vi "SNRPhaseNoiseStructure_ChangePowerFreq.vi"(7 "band":T1 {"stop frequency (Hz)" format="%.2f"; "start frequency (Hz)" format="%.2f"}, 8 "Analyze SNR Input":T2={"Pins"=["Xout"], "Published Data Id"=[], "frequency range"={"start frequency"=-1.0, "stop frequency"=-1.0}}, 9 "RFSG Input":T3={"LO configure setting"={"Carrier Frequency (Hz)"=5180000000.0, "Power Level(dBm)"=-10.0, "External Attenuation (dB)"=0.0}, "Port"=""} {"LO configure setting"."Carrier Frequency (Hz)" format="%#_6p"}, 10 "Scope Input":T4={"Min. Sample Rate"=1000000.0, "Min Record Length"=1000, "Vertical Coupling"=1, "Vertical Range (V)"=2.0, "Pins"=["Xout"]} {"Vertical Range (V)" format="%_3g"; "Vertical Coupling" items=["AC", "DC", "Ground"]; "Min. Sample Rate" format="%#_6p"}, 11 "Semiconductor Module Context":T5) -> (0 "error out":errorcluster)   [LabVIEW 2014]
uses:
  <vilib>/NI_TestStand_SemiconductorModule/NI_TestStand_Semiconductor_Module.lvlibp/PinMap/General/SemiconductorModuleContext.ctl
  Control/Scope Input.ctl
  Control/RFSG Input.ctl
  Control/Digitizier Analyze Input.ctl
  Control/Quene Type_Digitizer.ctl
  <vilib>/NI_TestStand_SemiconductorModule/NI_TestStand_Semiconductor_Module.lvlibp/PinMap/RF/RFPM/PinToNIRFPMSessions.vi
  <vilib>/NI_TestStand_SemiconductorModule/NI_TestStand_Semiconductor_Module.lvlibp
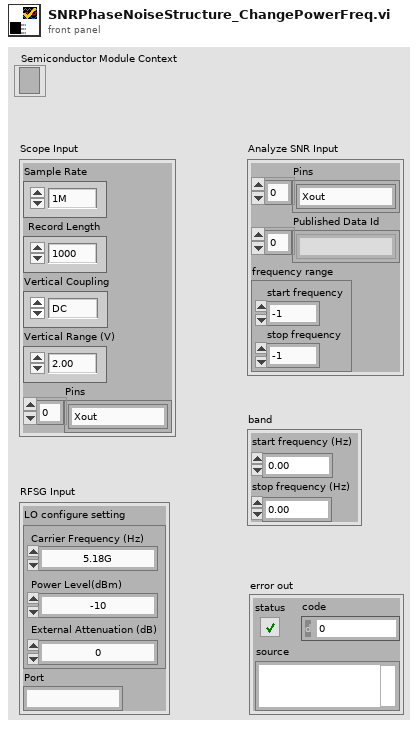
[diagram p1: front panel]
types:
  T1 = cluster{"start frequency (Hz)":dbl, "stop frequency (Hz)":dbl}
  T2 = typedef "Digitizier Analyze Input.ctl" = cluster{"Pins":string[], "Published Data Id":string[], "frequency range":cluster{"start frequency":dbl, "stop frequency":dbl}}
  T3 = typedef "RFSG Input.ctl" = cluster{"LO configure setting":cluster{"Carrier Frequency (Hz)":dbl, "Power Level(dBm)":dbl, "External Attenuation (dB)":dbl}, "Port":string}
  T4 = typedef "Scope Input.ctl" = cluster{"Min. Sample Rate":dbl, "Min Record Length":i32, "Vertical Coupling":i32, "Vertical Range (V)":dbl, "Pins":string[]}
  T5 = typedef "NI_TestStand_Semiconductor_Module.lvlibp/SemiconductorModuleContext.ctl" = refnum<k7>
  T6 = typedef "Quene Type_Digitizer.ctl" = cluster{"Actiion":enum16{"Exit", "Analyze"}, "Waveform Data":waveform(dbl)[], "Semiconductor Module Context":T5, "error constant":errorcluster}
  T7 = cluster{"Carrier Frequency (Hz)":dbl, "Power Level(dBm)":dbl, "External Attenuation (dB)":dbl}
  T8 = cluster{"start frequency":dbl, "stop frequency":dbl}
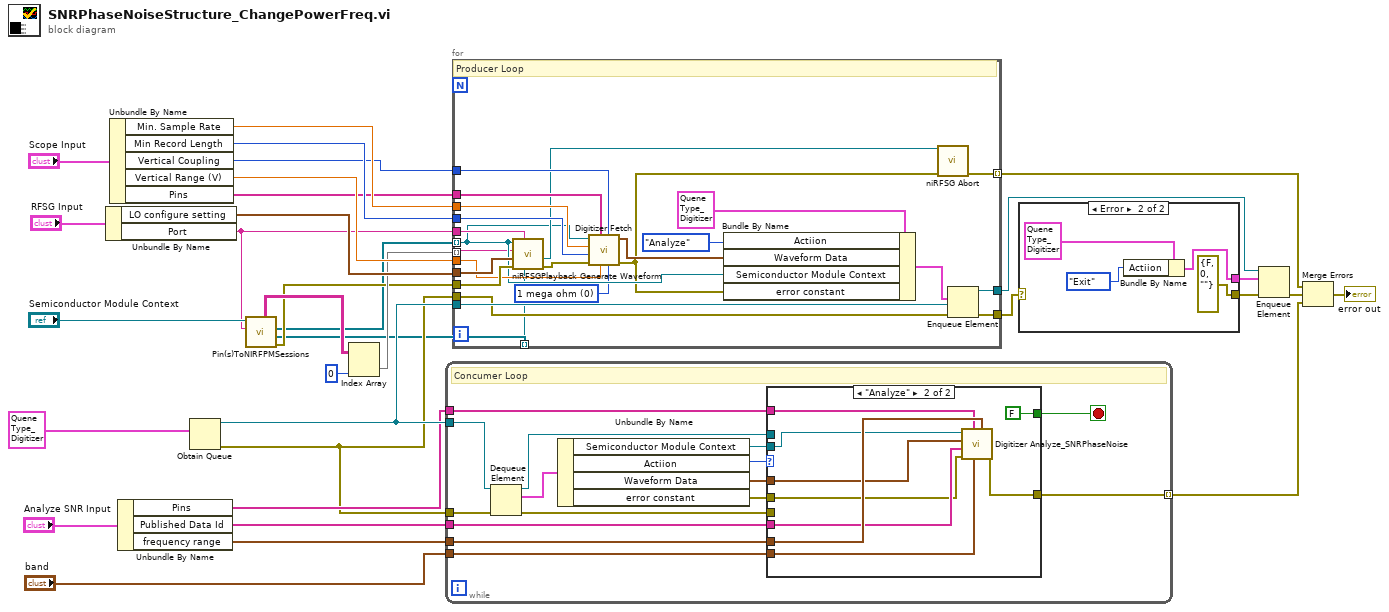
[diagram p0: block diagram]
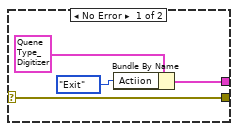
[diagram p2: hidden frame]
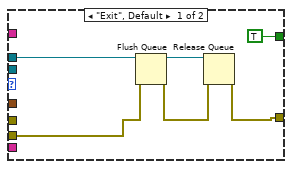
[diagram p3: hidden frame]
diagram:
  n1 = Unbundle By Name("RFSG Input") -> ("LO configure setting"=w30:T7, "Port"=w1:string)
  n2 = Unbundle By Name("Scope Input") -> ("Min. Sample Rate"=w28:dbl, "Min Record Length"=w27:i32, "Vertical Coupling"=w25:i32, "Vertical Range (V)"=w26:dbl, "Pins"=w24:string[])
  n3 = Unbundle By Name("Analyze SNR Input") -> ("Pins"=w18:string[], "Published Data Id"=w19:string[], "frequency range"=w20:T8)
  n4 = Obtain Queue(element data type=T6 {"Actiion"=enum."Analyze", "Waveform Data"=[], "Semiconductor Module Context"=refnum, "error constant"={"status"=FALSE, "code"=0, "source"=""}}) -> (queue out=w22:refnum<queue>, error out=w13:errorcluster)  [unwired: 4 in, 1 out]
  n5 = call-poly <vilib>:"Pin(s)ToNIRFPMSessions.vi"("Pin"=w1, "Semiconductor Module Context"="Semiconductor Module Context") -> ("error out"=w4:errorcluster, "Instrument Sessions"=w2:refnum<k15>[], "Semiconductor Module Contexts"=w3:refnum<k7>[], "Ports List"=w7:string[][])  [unwired: 4 in, 2 out]
  n6 = Index Array(array=w7, index (col)=0) -> (element=w6:string[])  [unwired: 1 in]
  n7 = while {
    tunnel: w22 -> [w47]
    tunnel: w20 -> [w41]
    tunnel: w19 -> [w40]
    tunnel: w18 -> [w39]
    tunnel: w13 -> [w46]
    tunnel: [w36] -> w15 mode=indexing
    tunnel: "band" -> [w35]
    stop <- w43 stop-if-true
    # "Concumer Loop"
    n8 = Dequeue Element(queue=w47, error in (no error)=w46) -> (queue out=w38:refnum<queue>, element=w45:T6, error out=w37:errorcluster)  [unwired: 1 in, 1 out]
    n9 = Unbundle By Name(w45) -> ("Semiconductor Module Context"=w34:T5, "Actiion"=w44:enum16{"Exit", "Analyze"}, "Waveform Data"=w42:waveform(dbl)[], "error constant"=w33:errorcluster)
    n10 = case shown="\"Analyze\"" w44 {
      tunnel: [TRUE FALSE] -> w43
      tunnel: w34 -> [_ w57]
      tunnel: w42 -> [_ w58]
      tunnel: w41 -> [_ w61]
      tunnel: w40 -> [_ w60]
      tunnel: w39 -> [_ w59]
      tunnel: w38 -> [w50 _]
      tunnel: w37 -> [w49 _]
      tunnel: [w48 w56] -> w36
      tunnel: w35 -> [_ w55]
      tunnel: w33 -> [_ w54]
      frame "Exit", Default {
        n11 = Flush Queue(queue=w50, error in (no error)=w49) -> (queue out=w52:refnum<queue>, error out=w51:errorcluster)  [unwired: 1 out]
        n12 = Release Queue(queue=w52, error in (no error)=w51) -> (error out=w48:errorcluster)  [unwired: 1 in, 2 out]
      }
      frame "Analyze" {
        n13 = call "Digitizer Analyze_SNRPhaseNoise.vi"("frequency range"=w61, "band"=w55, "Pins"=w59, "error in"=w54, "Published Data Id"=w60, "Waveform Data In"=w58, "Semiconductor Module Context"=w57) -> ("error out"=w56:errorcluster)  [unwired: 3 in]
      }
    }
  }
  n14 = for {
    tunnel: w3 -> [w67] mode=indexing
    tunnel: w30 -> [w85]
    tunnel: w1 -> [w84]
    tunnel: w28 -> [w83]
    tunnel: w27 -> [w82]
    tunnel: w26 -> [w80]
    tunnel: w25 -> [w79]
    tunnel: w24 -> [w78]
    tunnel: w22 -> [w77]
    tunnel: [w71] -> w23
    tunnel: w4 -> [w86]
    tunnel: [w69] -> w14 mode=indexing
    tunnel: w13 -> [w70]
    tunnel: [w72] -> w12
    tunnel: w6 -> [w66] mode=indexing
    tunnel: w2 -> [w65] mode=indexing
    w64 = u32 0 items=["1 mega ohm"=0, "50 ohms"=2] ("input impedance")
    # "Producer Loop"
    n15 = call "niRFSGPlayback Generate Waveform.vi"("instrument handle"=w65, "Port"=w84, "error in (no error)"=w86, "LO configure setting"=w85, "TX port"=w66, "TSM Context"=w67) -> ("error out"=w81:errorcluster, "instrument handle out"=w68:refnum<k15>)  [unwired: 4 in]
    n16 = call "Digitizer Fetch.vi"("input impedance"=w64, "Vertical Coupling"=w79, "Vertical Range (V)"=w80, "Pins"=w78, "error in (no error)"=w81, "Min Record Length"=w82, "Min. Sample Rate"=w83, "Semiconductor Module Context"=w67) -> ("error out"=w63:errorcluster, "Waveform Data Out"=w75:waveform(dbl)[])  [unwired: 2 in]
    n17 = Bundle By Name(cluster=T6 {"Actiion"=enum."Exit", "Waveform Data"=[], "Semiconductor Module Context"=refnum, "error constant"={"status"=FALSE, "code"=0, "source"=""}}, "Actiion"=enum16{"Exit", "Analyze"}."Analyze", "Waveform Data"=w75, "Semiconductor Module Context"=w67, "error constant"=w63) -> (w73:T6)
    n18 = call <instrlib>:"niRFSG Abort.vi"("instrument handle"=w68, "error in"=w63) -> ("error out"=w69:errorcluster)  [unwired: 12 in, 1 out]
    n19 = Enqueue Element(queue=w77, element=w73, error in (no error)=w70) -> (queue out=w71:refnum<queue>, error out=w72:errorcluster)  [unwired: 1 in, 1 out]
  }
  n20 = case shown="Error" w12 {
    selector: w12 -> [w87 _]
    tunnel: [w88 w91] -> w11
    tunnel: [w87 errorcluster {"status"=FALSE, "code"=0, "source"=""} ("error IO")] -> w10
    frame No Error {
      n21 = Bundle By Name(cluster=T6 {"Actiion"=enum."Analyze", "Waveform Data"=[], "Semiconductor Module Context"=refnum, "error constant"={"status"=FALSE, "code"=0, "source"=""}}, "Actiion"=enum16{"Exit", "Analyze"}."Exit") -> (w88:T6)
    }
    frame Error {
      n22 = Bundle By Name(cluster=T6 {"Actiion"=enum."Analyze", "Waveform Data"=[], "Semiconductor Module Context"=refnum, "error constant"={"status"=FALSE, "code"=0, "source"=""}}, "Actiion"=enum16{"Exit", "Analyze"}."Exit") -> (w91:T6)
    }
  }
  n23 = Enqueue Element(queue=w23, element=w11, error in (no error)=w10) -> (error out=w16:errorcluster)  [unwired: 1 in, 2 out]
  n24 = Merge Errors(w14, w16, w15) -> (→"error out":errorcluster)
